vi "Set Error.vi"(9 "Is Override":bool, 10 "Error":errorcluster, 11 "TEMPLATE Actor in":refnum<class "TEMPLATE Actor.lvclass">) -> (3 "TEMPLATE Actor out":refnum<class "TEMPLATE Actor.lvclass">)   [LabVIEW 2020, in "_Template.lvlib" / "Templates.lvlib" / "TEMPLATE Actor.lvlib" / "TEMPLATE Actor.lvclass"]
uses:
  TEMPLATE Actor.lvclass
  TEMPLATE Actor.lvclass/TEMPLATE Actor.ctl
  jettl/jettl/Actor/Actor/Actor.lvclass
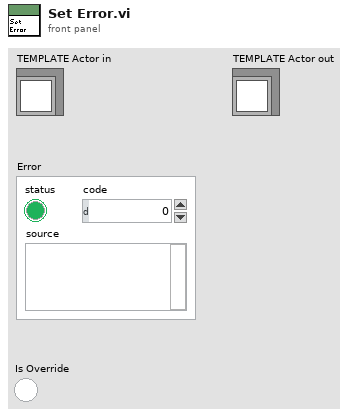
[diagram p1: front panel]
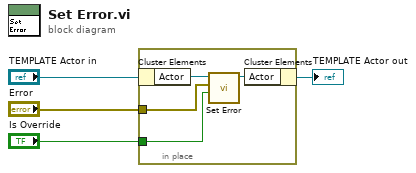
[diagram p0: block diagram]
diagram:
  n1 = in-place {
    in-place-border: "Error" -> [w6]
    in-place-border: "Is Override" -> [w5]
    n2 = in-place-cluster #1("TEMPLATE Actor in") -> ("Actor"=w8:refnum<class "Actor.lvclass">)
    n3 = call-dynamic "Set Error.vi"("Is Override"=w5, "Error"=w6, "Actor in"=w8) -> ("Actor out"=w7:refnum<class "Actor.lvclass">)  [unwired: 8 in]
    n4 = in-place-cluster #1("Actor"=w7) -> (→"TEMPLATE Actor out":refnum<class "TEMPLATE Actor.lvclass">)
  }
